vi "ex_1_ES_main.vi"() -> ()   [LabVIEW 2020]
panel:
  out "To be moved":string
  in  "Sound intensity: MAX":dbl=100.0
  in  "Sound intensity: MIN":dbl
  out "Limit exceeded?":bool
  in  "Stop Button":bool
  in  "Sound intensity [dB]":dbl(slide) scale=0.0..100.0
  # "85 dB"
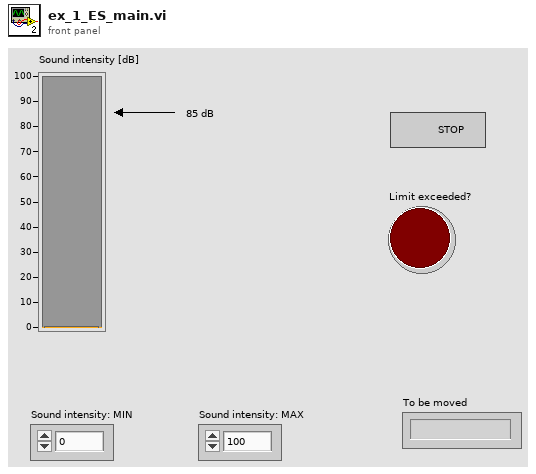
[diagram p1: front panel]
types:
  T1 = typedef "LVPoint32TypeDef.ctl" = cluster{"Horizontal":i32, "Vertical":i32}
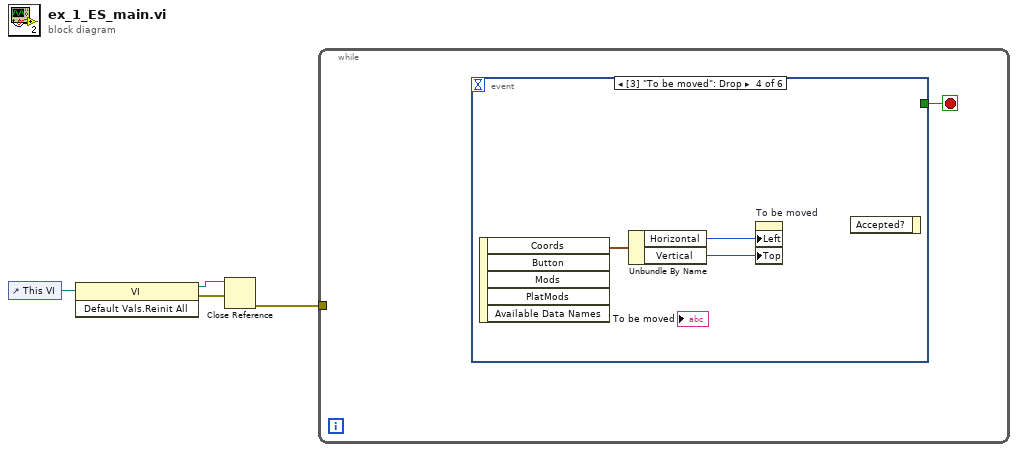
[diagram p0: block diagram]
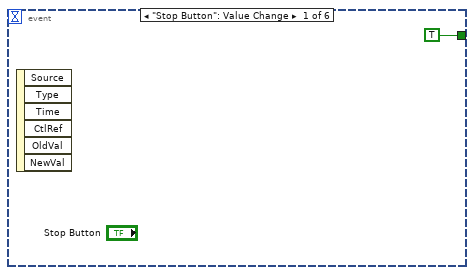
[diagram p2: hidden frame]
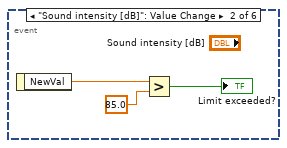
[diagram p3: hidden frame]
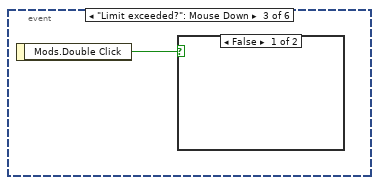
[diagram p4: hidden frame]
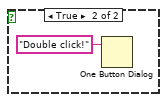
[diagram p5: hidden frame]
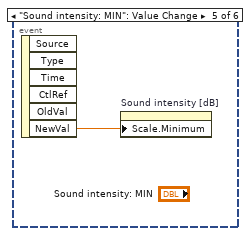
[diagram p6: hidden frame]
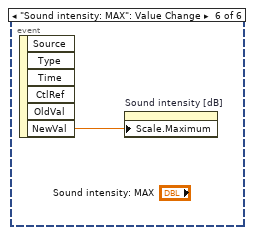
[diagram p7: hidden frame]
diagram:
  n1 = control-ref of="This VI"() -> (w4:refnum<vi>)
  n2 = invoke class="VI" method="Default Vals.Reinit All"(reference=w4) -> (reference out=w3:refnum<vi>, error out=w2:errorcluster)  [unwired: 2 in, 1 out]
  n3 = Close Reference(reference=w3, error in (no error)=w2) -> (error out=w1:errorcluster)
  n4 = while {
    tunnel: w1 -> [_]
    stop <- w5 stop-if-true
    n5 = event shown="[3] \"To be moved\": Drop" {
      selector: _ -> [_ _ _ _ _ _]
      dyn-events: _ -> [_ _ _ _ _ _]
      timeout: _ -> [_ _ _ _ _ _]
      tunnel: [TRUE _ _ _ _ _] -> w5
      event "Stop Button": Value Change {
        n6 = event-data() -> ()  [unwired: 1 in, 6 out]
      }
      event "Sound intensity [dB]": Value Change {
        n7 = event-data() -> ("NewVal"=w9:dbl)  [unwired: 1 in]
        n8 = Greater?(x=w9, y=85.0) -> (0:→"Limit exceeded?":bool)
      }
      event "Limit exceeded?": Mouse Down {
        n9 = event-data() -> ("Mods.Double Click"=w10:bool)  [unwired: 1 in]
        n10 = case shown="False" w10 {
          frame False {
          }
          frame True {
            n11 = One Button Dialog(message="Double click!") -> ()  [unwired: 1 in, 1 out]
          }
        }
      }
      event "To be moved": Drop {
        n12 = event-data() -> ("Coords"=w14:T1)  [unwired: 1 in, 4 out]
        n13 = Unbundle By Name(w14) -> ("Horizontal"=w13:i32, "Vertical"=w12:i32)
        n14 = property on="To be moved" class="Str"("Left"=w13, "Top"=w12) -> ()  [unwired: 2 in, 2 out]
        n15 = event-data() -> ()  [unwired: 2 in, 1 out]
      }
      event "Sound intensity: MIN": Value Change {
        n16 = event-data() -> ("NewVal"=w15:dbl)  [unwired: 1 in, 5 out]
        n17 = property on="Sound intensity [dB]" class="Slide (strict)"("Scale.Minimum"=w15) -> ()  [unwired: 2 in, 2 out]
      }
      event "Sound intensity: MAX": Value Change {
        n18 = event-data() -> ("NewVal"=w16:dbl)  [unwired: 1 in, 5 out]
        n19 = property on="Sound intensity [dB]" class="Slide (strict)"("Scale.Maximum"=w16) -> ()  [unwired: 2 in, 2 out]
      }
    }
  }
